vi "Close Plotter Session.vi"(8 "error in (no error)":errorcluster, 11 "PythonPlotter in":refnum<class "PythonPlotter.lvclass">) -> (0 "error out":errorcluster, 3 "PythonPlotter out":refnum<class "PythonPlotter.lvclass">)   [LabVIEW 2024, in "PythonPlotter.lvclass"]
uses:
  PythonPlotter.lvclass
  PythonPlotter.lvclass/PythonPlotter.ctl
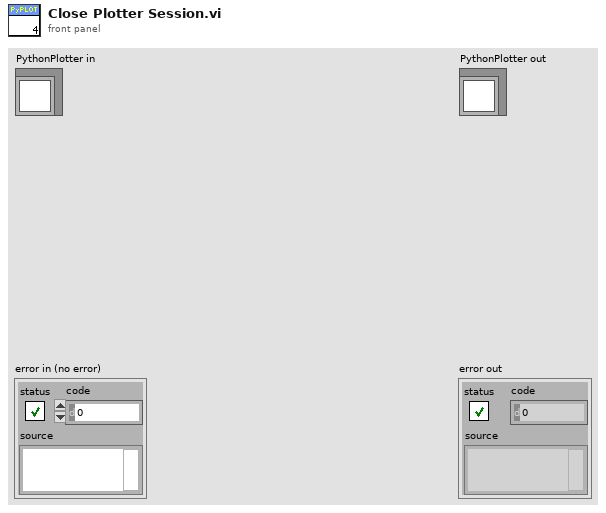
[diagram p1: front panel]
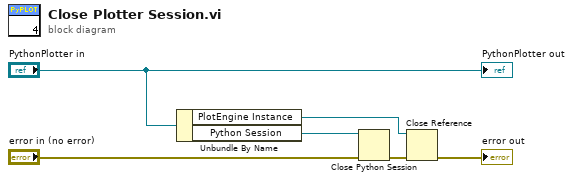
[diagram p0: block diagram]
diagram:
  n1 = Unbundle By Name("PythonPlotter in") -> ("PlotEngine Instance"=w4:refnum<k38>, "Python Session"=w5:refnum<k35>)
  n2 = Close Python Session(session in=w5, error in="error in (no error)") -> (11:w3:errorcluster)
  n3 = Close Reference(reference=w4, error in (no error)=w3) -> (error out=→"error out":errorcluster)
  "PythonPlotter out" <- "PythonPlotter in"
